vi "Frame number to Voltage.vi"(5 "Channel N":i16, 7 "SIM Frame N":i16, 8 "Voltages":dbl[][](array[numeric]) format="%0.3f", 9 "Frame count":i16, 10 "Current Channel":i16, 11 "Current V":i16) -> (0 "Final frame?":bool, 1 "V":dbl, 2 "Channel out":i16, 3 "Voltage out":i16, 4 "First frame?":bool)   [LabVIEW 2012]
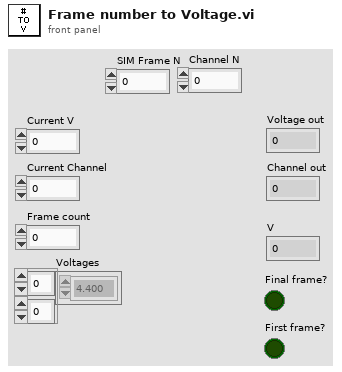
[diagram p1: front panel]
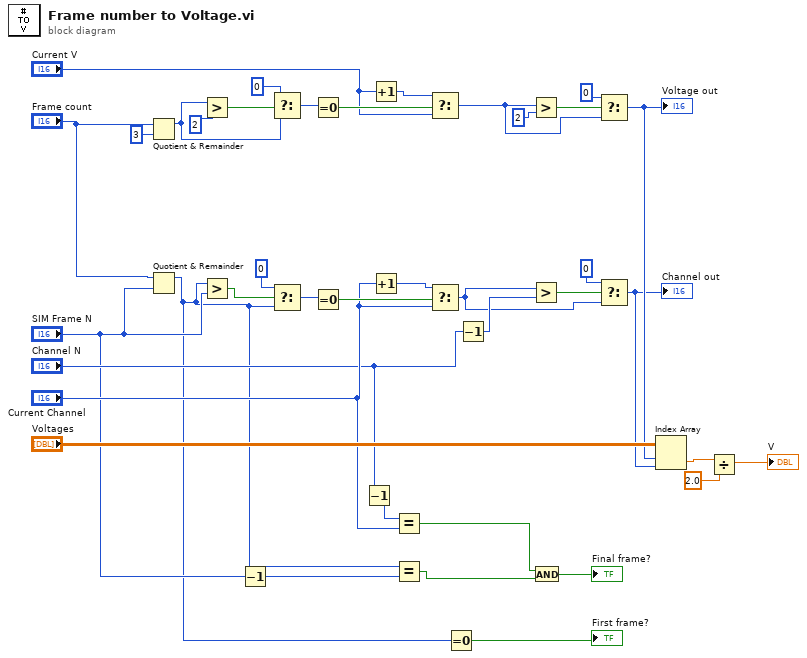
[diagram p0: block diagram]
diagram:
  n1 = Quotient & Remainder(x="Frame count", y=i16 3) -> (x-y*floor(x/y)=w28:i16)  [unwired: 1 out]
  n2 = Quotient & Remainder(x="Frame count", y="SIM Frame N") -> (x-y*floor(x/y)=w2:i16)  [unwired: 1 out]
  n3 = Greater?(x=w28, y=i16 2) -> (0:w37:bool)
  n4 = Greater?(x=w2, y="SIM Frame N") -> (0:w27:bool)
  n5 = Decrement(x="SIM Frame N") -> (x-1=w5:i16)
  n6 = Select(t=i16 0, s=w37, f=w28) -> (s? t:f=w35:i16)
  n7 = Select(t=i16 0, s=w27, f=w2) -> (s? t:f=w21:i16)
  n8 = Equal To 0?(x=w35) -> (x = 0?=w34:bool)
  n9 = Equal To 0?(x=w21) -> (x = 0?=w20:bool)
  n10 = Decrement(x="Channel N") -> (x-1=w4:i16)
  n11 = Increment(x="Current V") -> (x+1=w33:i16)
  n12 = Increment(x="Current Channel") -> (x+1=w25:i16)
  n13 = Equal?(x=w4, y="Current Channel") -> (x = y?=w8:bool)
  n14 = Equal?(x=w2, y=w5) -> (x = y?=w7:bool)
  n15 = Select(t=w33, s=w34, f="Current V") -> (s? t:f=w19:i16)
  n16 = Select(t=w25, s=w20, f="Current Channel") -> (s? t:f=w18:i16)
  n17 = Equal To 0?(x=w2) -> (x = 0?=→"First frame?":bool)
  n18 = Decrement(x="Channel N") -> (x-1=w24:i16)
  n19 = Greater?(x=w19, y=i16 2) -> (0:w31:bool)
  n20 = Greater?(x=w18, y=w24) -> (0:w23:bool)
  n21 = And(x=w8, y=w7) -> (x .and. y?=→"Final frame?":bool)
  n22 = Select(t=i16 0, s=w31, f=w19) -> (s? t:f=w16:i16)
  "Voltage out" <- w16
  n23 = Select(t=i16 0, s=w23, f=w18) -> (s? t:f=w15:i16)
  "Channel out" <- w15
  n24 = Index Array(array="Voltages", index (row)=w16, index (col)=w15) -> (element=w14:dbl)
  n25 = Divide(x=w14, y=2.0) -> (x/y=→"V":dbl)
